vi "MIDI Config.vi"(4 "MIDI device:":i32) -> (1 "Selected device":i32=1)   [LabVIEW 2016]
panel:
  in  "stop 2":bool
  in  "stop":bool
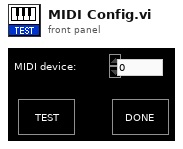
[diagram p1: front panel]
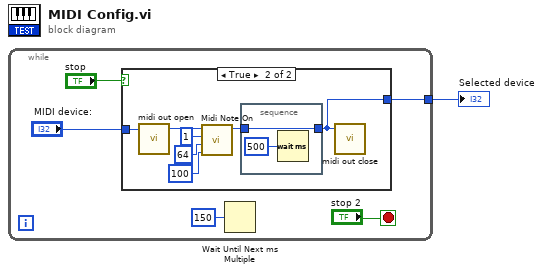
[diagram p0: block diagram]
diagram:
  n1 = while {
    tunnel: [w2] -> w1
    stop <- "stop 2" stop-if-true
    n2 = case shown="True" "stop" {
      tunnel: "MIDI device:" -> [w7 w14]
      tunnel: [w7 w8] -> w2
      frame False {
      }
      frame True {
        n3 = call "midi out open.vi"("UDeviceID"=w14) -> ("Hmidiout handle"=w13:i32)  [unwired: 5 in, 1 out]
        n4 = call "Midi Note On.vi"("Volume"=100, "Note"=64, "Channel"=1 ("channel"), "MIDI handle"=w13) -> ("Duplicate MIDI handle"=w12:i32)  [unwired: 2 in, 1 out]
        n5 = stacked-sequence {
          tunnel: w12 -> [w16]
          tunnel: [w16] -> w8
          frame #0 {
            n6 = Wait (ms)(milliseconds to wait=u32 500) -> ()  [unwired: 1 out]
          }
        }
        n7 = call "midi out close.vi"("MIDI output handle"=w8) -> ()  [unwired: 6 in, 1 out]
      }
    }
    n8 = Wait Until Next ms Multiple(millisecond multiple=u32 150) -> ()  [unwired: 1 out]
  }
  "Selected device" <- w1
